vi "Execute.vi"(5 "SleepTerminalArray":refnum<vi>, 6 "ExeRef":refnum<vi>, 7 "ActiveTerminalArray":refnum<vi>, 8 "error in (no error)":errorcluster, 9 "Json_In":string, 10 "VariableRef":T2, 11 "Info":T1) -> (0 "Error Out":errorcluster, 1 "NumResultArray":dbl[](array[numeric]), 2 "StrResultArray":string[](array[string]), 3 "StrResult":string, 4 "NumResult":dbl)   [LabVIEW 2018, in "Number.lvlib"]
uses:
  Number.lvlib
  <userlib>/_OpenG.lib/dictionary/dictionary.llb/Dictionary Object RefNum__ogtk.ctl
  <userlib>/_OpenG.lib/dictionary/dictionary.llb/Dictionary Object RefNum - Enum__ogtk.ctl
  <vilib>/addons/_JKI.lib/Serialization/JSON/JKI JSON Serialization.lvlib
  <vilib>/gmath/NI_Gmath.lvlib
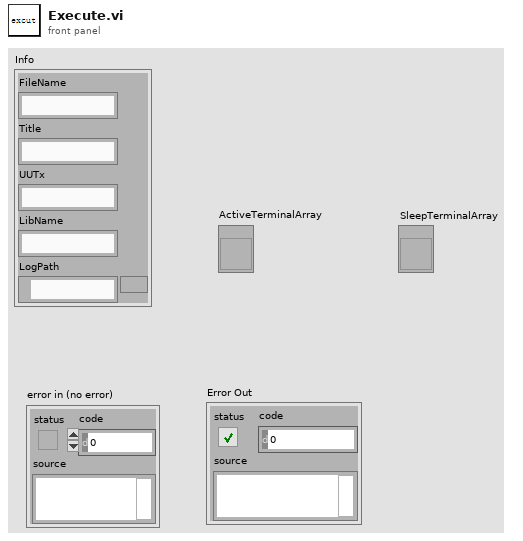
[diagram p1: front panel]
types:
  T1 = cluster{"FileName":string, "Title":string, "UUTx":string, "LibName":string, "LogPath":path}
  T2 = typedef "Dictionary Object RefNum__ogtk.ctl" = refnum<k1>
  T3 = cluster{"InitialNumber":cluster{"json":cluster{"Method":string, "InitialNum":dbl}}, "RandomNumber":cluster{"json":cluster{"Method":string, "Seed":dbl}}, "CalculateNumber":cluster{"json":cluster{"Method":string, "Type":string, "NumxVar":string, "NumyVar":string, "Formula":string}}, "CompareNumber":cluster{"json":cluster{"Method":string, "Type":string, "NumxVar":string, "NumyVar":string}}}
  T4 = cluster{"json":cluster{"Method":string, "InitialNum":dbl}}
  T5 = cluster{"json":cluster{"Method":string, "Seed":dbl}}
  T6 = cluster{"json":cluster{"Method":string, "Type":string, "NumxVar":string, "NumyVar":string, "Formula":string}}
  T7 = cluster{"json":cluster{"Method":string, "Type":string, "NumxVar":string, "NumyVar":string}}
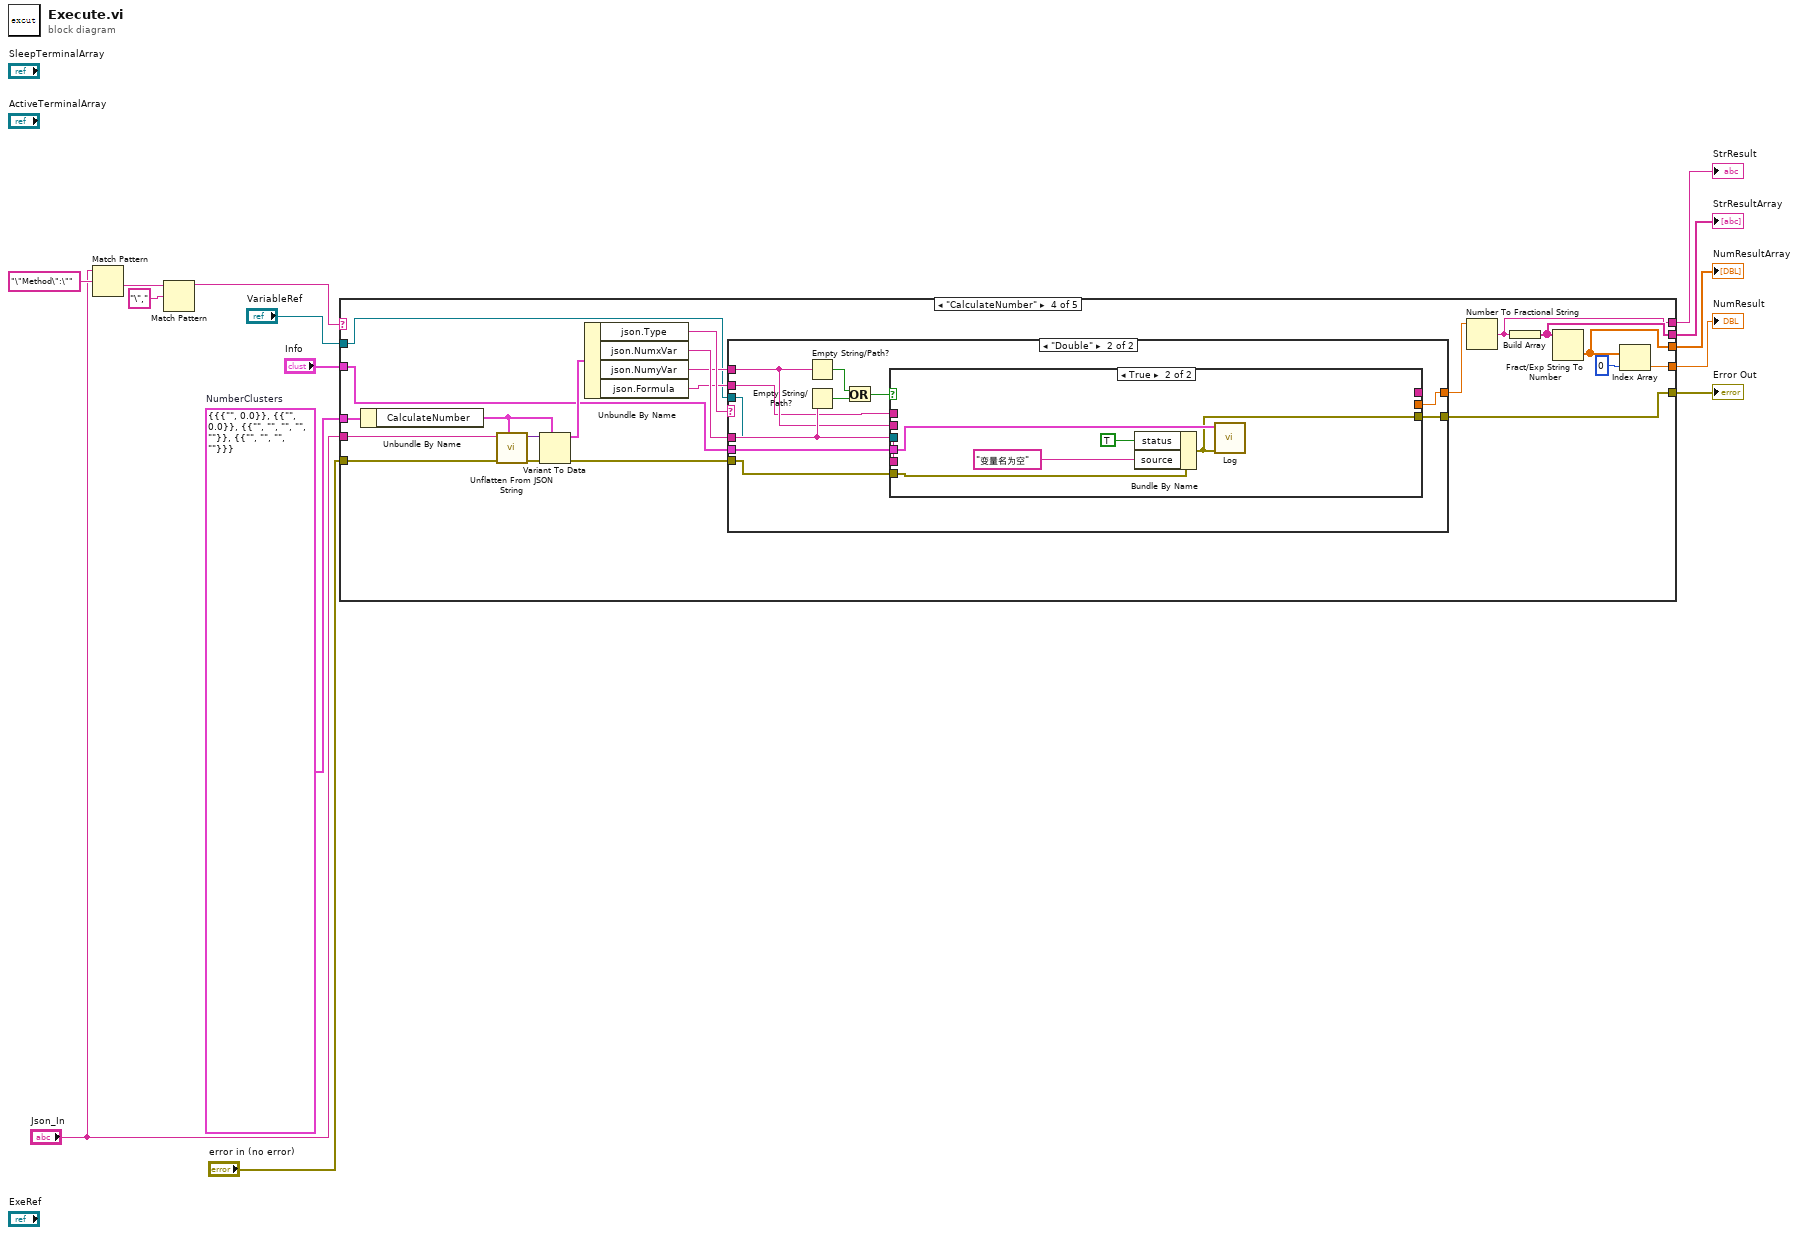
[diagram p0: block diagram]
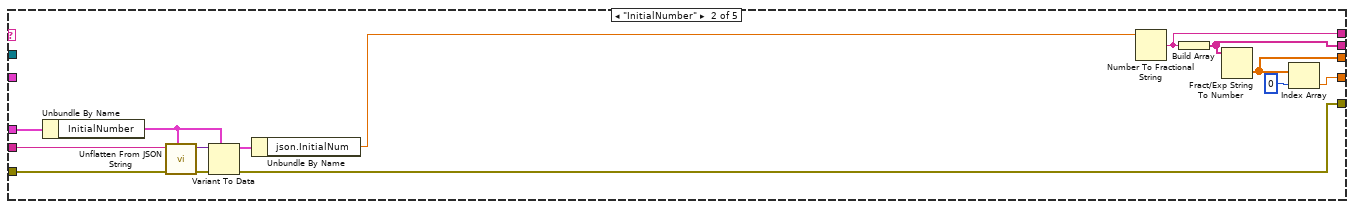
[diagram p3: hidden frame]
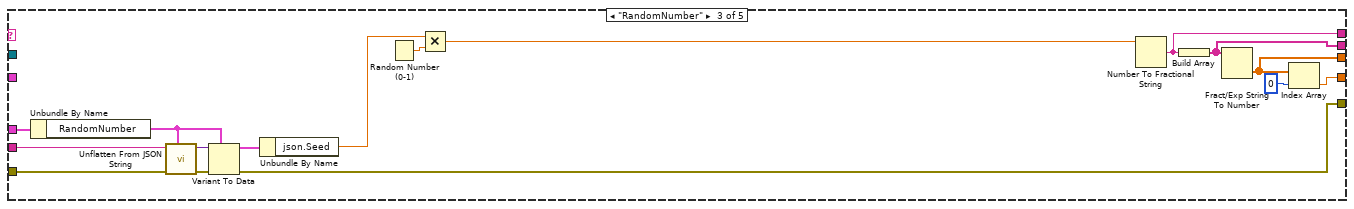
[diagram p4: hidden frame]
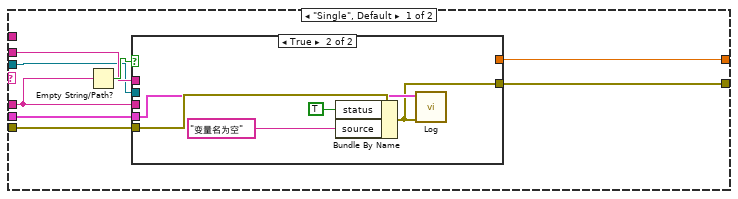
[diagram p5: hidden frame]
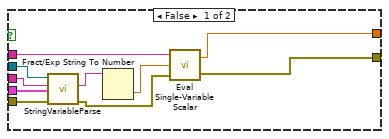
[diagram p6: hidden frame]
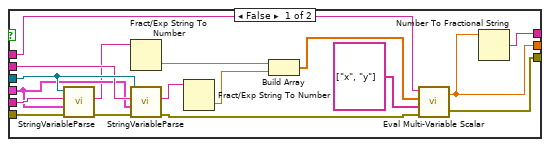
[diagram p7: hidden frame]
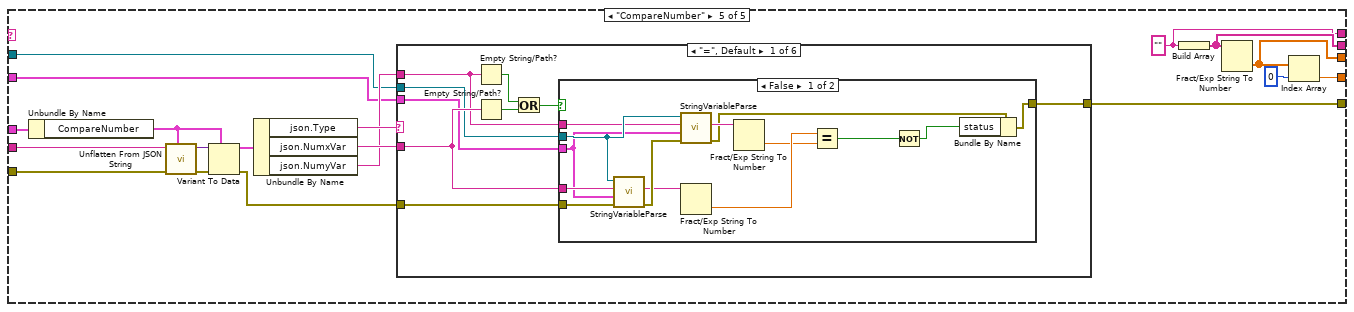
[diagram p8: hidden frame]
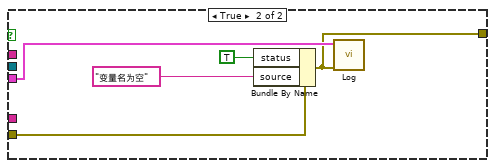
[diagram p9: hidden frame]
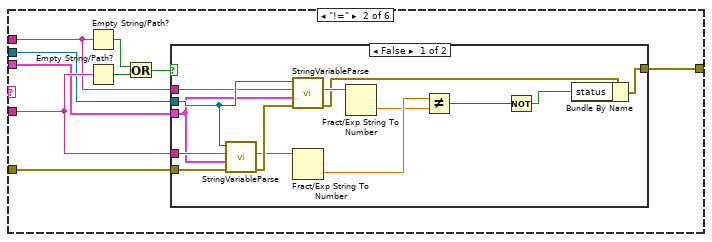
[diagram p10: hidden frame]
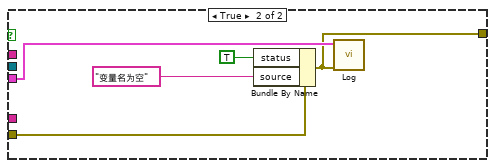
[diagram p11: hidden frame]
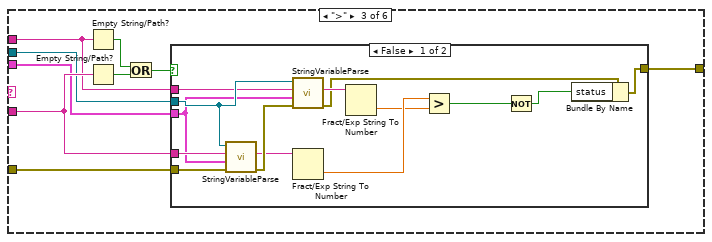
[diagram p12: hidden frame]
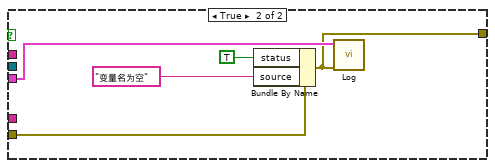
[diagram p13: hidden frame]
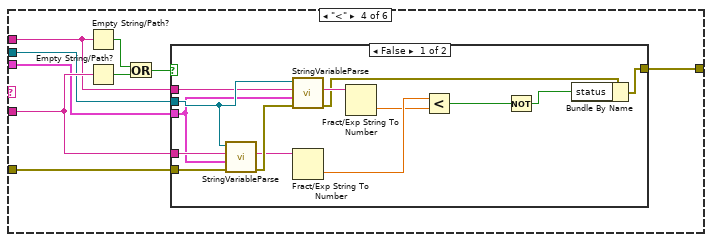
[diagram p14: hidden frame]
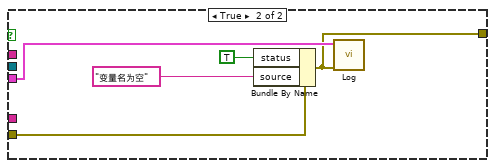
[diagram p15: hidden frame]
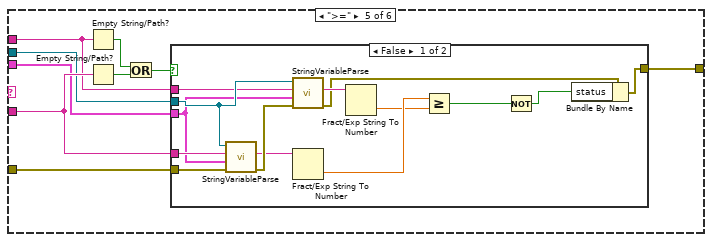
[diagram p16: hidden frame]
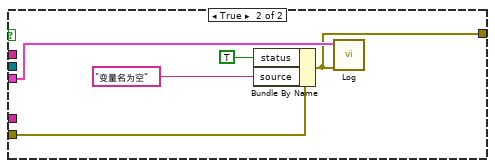
[diagram p17: hidden frame]
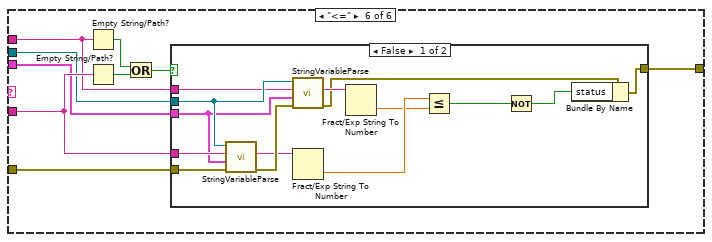
[diagram p18: hidden frame]
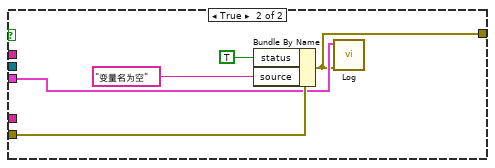
[diagram p19: hidden frame]
diagram:
  w1 = T3 {"InitialNumber"={"json"={"Method"="", "InitialNum"=0.0}}, "RandomNumber"={"json"={"Method"="", "Seed"=0.0}}, "CalculateNumber"={"json"={"Method"="", "Type"="", "NumxVar"="", "NumyVar"="", "Formula"=""}}, "CompareNumber"={"json"={"Method"="", "Type"="", "NumxVar"="", "NumyVar"=""}}}  # NumberClusters
  n1 = Match Pattern(string="Json_In", regular expression="\"Method\":\"") -> (after substring=w4:string)  [unwired: 1 in, 3 out]
  n2 = Match Pattern(string=w4, regular expression="\",") -> (before substring=w2:string)  [unwired: 1 in, 3 out]
  n3 = case shown="\"CalculateNumber\"" w2 {
    tunnel: "Json_In" -> [_ w26 w42 w63 w138]
    tunnel: [w15 w18 w34 w46 w124] -> w14
    tunnel: "error in (no error)" -> [w15 w25 w41 w62 w137]
    tunnel: [_ w17 w33 w47 w123] -> w12
    tunnel: "VariableRef" -> [_ _ _ w49 w125]
    tunnel: [_ w16 w32 w56 w131] -> w11
    tunnel: [_ w21 w37 w59 w134] -> w10
    tunnel: [_ w23 w39 w61 w136] -> w9
    tunnel: "Info" -> [_ _ _ w50 w126]
    tunnel: w1 -> [_ w20 w36 w58 w133]
    frame Default {
    }
    frame "InitialNumber" {
      n4 = Unbundle By Name(w20) -> ("InitialNumber"=w19:T4)
      n5 = call <vilib>:"Unflatten From JSON String.vi"("Type and Defaults"=w19, "error in (no error)"=w25, "JSON String"=w26) -> ("error out"=w28:errorcluster, "Variant"=w29:variant)  [unwired: 7 in]
      n6 = Variant To Data(error in=w28, type=w19, Variant=w29) -> (data=w27:T4, error out=w18:errorcluster)
      n7 = Unbundle By Name(w27) -> ("json.InitialNum"=w24:dbl)
      n8 = Number To Fractional String(number=w24) -> (F-format string=w17:string)  [unwired: 3 in]
      n9 = Build Array(w17) -> (w16:string[])
      n10 = Fract/Exp String To Number(string=w16) -> (number=w23:dbl[])  [unwired: 3 in, 1 out]
      n11 = Index Array(array=w23, index=0) -> (element=w21:dbl)
    }
    frame "RandomNumber" {
      n12 = Unbundle By Name(w36) -> ("RandomNumber"=w35:T5)
      n13 = call <vilib>:"Unflatten From JSON String.vi"("Type and Defaults"=w35, "error in (no error)"=w41, "JSON String"=w42) -> ("error out"=w44:errorcluster, "Variant"=w45:variant)  [unwired: 7 in]
      n14 = Variant To Data(error in=w44, type=w35, Variant=w45) -> (data=w43:T5, error out=w34:errorcluster)
      n15 = Unbundle By Name(w43) -> ("json.Seed"=w40:dbl)
      n16 = Random Number (0-1)() -> (number: 0 to 1=w30:dbl)
      n17 = Multiply(x=w40, y=w30) -> (x*y=w31:dbl)
      n18 = Number To Fractional String(number=w31) -> (F-format string=w33:string)  [unwired: 3 in]
      n19 = Build Array(w33) -> (w32:string[])
      n20 = Fract/Exp String To Number(string=w32) -> (number=w39:dbl[])  [unwired: 3 in, 1 out]
      n21 = Index Array(array=w39, index=0) -> (element=w37:dbl)
    }
    frame "CalculateNumber" {
      n22 = Unbundle By Name(w58) -> ("CalculateNumber"=w57:T6)
      n23 = call <vilib>:"Unflatten From JSON String.vi"("Type and Defaults"=w57, "error in (no error)"=w62, "JSON String"=w63) -> ("error out"=w65:errorcluster, "Variant"=w66:variant)  [unwired: 7 in]
      n24 = Variant To Data(error in=w65, type=w57, Variant=w66) -> (data=w64:T6, error out=w54:errorcluster)
      n25 = Unbundle By Name(w64) -> ("json.Type"=w55:string, "json.NumxVar"=w53:string, "json.NumyVar"=w52:string, "json.Formula"=w51:string)
      n26 = case shown="\"Double\"" w55 {
        tunnel: w54 -> [w74 w100]
        tunnel: [w73 w99] -> w46
        tunnel: w53 -> [w72 w98]
        tunnel: [w71 w97] -> w48
        tunnel: w52 -> [_ w93]
        tunnel: w51 -> [w69 w92]
        tunnel: w50 -> [w68 w91]
        tunnel: w49 -> [w67 w90]
        frame "Single", Default {
          n27 = Empty String/Path?(string/path=w72) -> (empty?=w70:bool)
          n28 = case shown="True" w70 {
            tunnel: w74 -> [w78 w89]
            tunnel: [w84 w85] -> w73
            tunnel: w72 -> [w79 _]
            tunnel: [w81 _] -> w71
            tunnel: w69 -> [w83 _]
            tunnel: w68 -> [w75 w87]
            tunnel: w67 -> [w80 _]
            frame False {
              n29 = call "StringVariableParse.vi"("error in"=w78, "Info"=w75, "in"=w79, "dictionary"=w80) -> ("error out"=w77:errorcluster, "out"=w76:string)  [unwired: 5 in, 1 out]
              n30 = Fract/Exp String To Number(string=w76) -> (number=w82:dbl)  [unwired: 3 in, 1 out]
              n31 = call <vilib>:"Eval Single-Variable Scalar.vi"("error in (no error)"=w77, "x value"=w82, "formula"=w83) -> ("error out"=w84:errorcluster, "y value"=w81:dbl)
            }
            frame True {
              n32 = Bundle By Name(cluster=w89, "status"=TRUE, "source"="变量名为空") -> (w85:errorcluster)
              n33 = call "Log.vi"("error in"=w85, "Info"=w87) -> ()  [unwired: 10 in]
            }
          }
        }
        frame "Double" {
          n34 = Empty String/Path?(string/path=w93) -> (empty?=w94:bool)
          n35 = Empty String/Path?(string/path=w98) -> (empty?=w96:bool)
          n36 = Or(x=w94, y=w96) -> (x .or. y?=w95:bool)
          n37 = case shown="True" w95 {
            tunnel: w100 -> [w105 w122]
            tunnel: [w112 w118] -> w99
            tunnel: w98 -> [w109 _]
            tunnel: [w110 _] -> _
            tunnel: [w111 _] -> w97
            tunnel: w93 -> [w107 _]
            tunnel: w92 -> [w117 _]
            tunnel: w91 -> [w106 w119]
            tunnel: w90 -> [w108 _]
            frame False {
              n38 = call "StringVariableParse.vi"("error in"=w105, "Info"=w106, "in"=w109, "dictionary"=w108) -> ("error out"=w104:errorcluster, "out"=w101:string)  [unwired: 5 in, 1 out]
              n39 = Fract/Exp String To Number(string=w101) -> (number=w115:dbl)  [unwired: 3 in, 1 out]
              n40 = call "StringVariableParse.vi"("error in"=w104, "Info"=w106, "in"=w107, "dictionary"=w108) -> ("error out"=w103:errorcluster, "out"=w102:string)  [unwired: 5 in, 1 out]
              n41 = Fract/Exp String To Number(string=w102) -> (number=w114:dbl)  [unwired: 3 in, 1 out]
              n42 = Build Array(w115, w114) -> (w113:dbl[])
              n43 = call <vilib>:"Eval Multi-Variable Scalar.vi"("error in (no error)"=w103, "Variables"=string[] ["x", "y"], "X Values"=w113, "formula"=w117) -> ("error out"=w112:errorcluster, "y value"=w111:dbl)
              n44 = Number To Fractional String(number=w111) -> (F-format string=w110:string)  [unwired: 3 in]
            }
            frame True {
              n45 = Bundle By Name(cluster=w122, "status"=TRUE, "source"="变量名为空") -> (w118:errorcluster)
              n46 = call "Log.vi"("error in"=w118, "Info"=w119) -> ()  [unwired: 10 in]
            }
          }
        }
      }
      n47 = Number To Fractional String(number=w48) -> (F-format string=w47:string)  [unwired: 3 in]
      n48 = Build Array(w47) -> (w56:string[])
      n49 = Fract/Exp String To Number(string=w56) -> (number=w61:dbl[])  [unwired: 3 in, 1 out]
      n50 = Index Array(array=w61, index=0) -> (element=w59:dbl)
    }
    frame "CompareNumber" {
      w123 = ""
      n51 = Unbundle By Name(w133) -> ("CompareNumber"=w132:T7)
      n52 = call <vilib>:"Unflatten From JSON String.vi"("Type and Defaults"=w132, "error in (no error)"=w137, "JSON String"=w138) -> ("error out"=w140:errorcluster, "Variant"=w141:variant)  [unwired: 7 in]
      n53 = Variant To Data(error in=w140, type=w132, Variant=w141) -> (data=w139:T7, error out=w129:errorcluster)
      n54 = Unbundle By Name(w139) -> ("json.Type"=w130:string, "json.NumxVar"=w128:string, "json.NumyVar"=w127:string)
      n55 = case shown="\"=\", Default" w130 {
        tunnel: w129 -> [w150 w178 w206 w234 w262 w290]
        tunnel: [w149 w177 w205 w233 w261 w289] -> w124
        tunnel: w128 -> [w148 w176 w204 w232 w260 w288]
        tunnel: w127 -> [w144 w172 w200 w228 w256 w284]
        tunnel: w126 -> [w143 w171 w199 w227 w255 w283]
        tunnel: w125 -> [w142 w170 w198 w226 w254 w282]
        frame "=", Default {
          n56 = Empty String/Path?(string/path=w144) -> (empty?=w145:bool)
          n57 = Empty String/Path?(string/path=w148) -> (empty?=w147:bool)
          n58 = Or(x=w145, y=w147) -> (x .or. y?=w146:bool)
          n59 = case shown="False" w146 {
            tunnel: w150 -> [w160 w169]
            tunnel: [w153 w165] -> w149
            tunnel: w148 -> [w164 _]
            tunnel: w144 -> [w162 _]
            tunnel: w143 -> [w161 w166]
            tunnel: w142 -> [w163 _]
            frame False {
              n60 = call "StringVariableParse.vi"("error in"=w160, "Info"=w161, "in"=w164, "dictionary"=w163) -> ("error out"=w159:errorcluster, "out"=w157:string)  [unwired: 5 in, 1 out]
              n61 = call "StringVariableParse.vi"("error in"=w159, "Info"=w161, "in"=w162, "dictionary"=w163) -> ("error out"=w152:errorcluster, "out"=w158:string)  [unwired: 5 in, 1 out]
              n62 = Fract/Exp String To Number(string=w157) -> (number=w156:dbl)  [unwired: 3 in, 1 out]
              n63 = Fract/Exp String To Number(string=w158) -> (number=w155:dbl)  [unwired: 3 in, 1 out]
              n64 = Equal?(x=w156, y=w155) -> (x = y?=w151:bool)
              n65 = Not(x=w151) -> (.not. x?=w154:bool)
              n66 = Bundle By Name(cluster=w152, "status"=w154) -> (w153:errorcluster)
            }
            frame True {
              n67 = Bundle By Name(cluster=w169, "status"=TRUE, "source"="变量名为空") -> (w165:errorcluster)
              n68 = call "Log.vi"("error in"=w165, "Info"=w166) -> ()  [unwired: 10 in]
            }
          }
        }
        frame "!=" {
          n69 = Empty String/Path?(string/path=w172) -> (empty?=w173:bool)
          n70 = Empty String/Path?(string/path=w176) -> (empty?=w175:bool)
          n71 = Or(x=w173, y=w175) -> (x .or. y?=w174:bool)
          n72 = case shown="False" w174 {
            tunnel: w178 -> [w188 w197]
            tunnel: [w181 w193] -> w177
            tunnel: w176 -> [w192 _]
            tunnel: w172 -> [w190 _]
            tunnel: w171 -> [w189 w194]
            tunnel: w170 -> [w191 _]
            frame False {
              n73 = call "StringVariableParse.vi"("error in"=w188, "Info"=w189, "in"=w192, "dictionary"=w191) -> ("error out"=w187:errorcluster, "out"=w185:string)  [unwired: 5 in, 1 out]
              n74 = call "StringVariableParse.vi"("error in"=w187, "Info"=w189, "in"=w190, "dictionary"=w191) -> ("error out"=w180:errorcluster, "out"=w186:string)  [unwired: 5 in, 1 out]
              n75 = Fract/Exp String To Number(string=w185) -> (number=w184:dbl)  [unwired: 3 in, 1 out]
              n76 = Fract/Exp String To Number(string=w186) -> (number=w183:dbl)  [unwired: 3 in, 1 out]
              n77 = Not Equal?(x=w184, y=w183) -> (x != y?=w179:bool)
              n78 = Not(x=w179) -> (.not. x?=w182:bool)
              n79 = Bundle By Name(cluster=w180, "status"=w182) -> (w181:errorcluster)
            }
            frame True {
              n80 = Bundle By Name(cluster=w197, "status"=TRUE, "source"="变量名为空") -> (w193:errorcluster)
              n81 = call "Log.vi"("error in"=w193, "Info"=w194) -> ()  [unwired: 10 in]
            }
          }
        }
        frame ">" {
          n82 = Empty String/Path?(string/path=w200) -> (empty?=w201:bool)
          n83 = Empty String/Path?(string/path=w204) -> (empty?=w203:bool)
          n84 = Or(x=w201, y=w203) -> (x .or. y?=w202:bool)
          n85 = case shown="False" w202 {
            tunnel: w206 -> [w216 w225]
            tunnel: [w209 w221] -> w205
            tunnel: w204 -> [w220 _]
            tunnel: w200 -> [w218 _]
            tunnel: w199 -> [w217 w222]
            tunnel: w198 -> [w219 _]
            frame False {
              n86 = call "StringVariableParse.vi"("error in"=w216, "Info"=w217, "in"=w220, "dictionary"=w219) -> ("error out"=w215:errorcluster, "out"=w213:string)  [unwired: 5 in, 1 out]
              n87 = call "StringVariableParse.vi"("error in"=w215, "Info"=w217, "in"=w218, "dictionary"=w219) -> ("error out"=w208:errorcluster, "out"=w214:string)  [unwired: 5 in, 1 out]
              n88 = Fract/Exp String To Number(string=w213) -> (number=w212:dbl)  [unwired: 3 in, 1 out]
              n89 = Fract/Exp String To Number(string=w214) -> (number=w211:dbl)  [unwired: 3 in, 1 out]
              n90 = Greater?(x=w212, y=w211) -> (0:w207:bool)
              n91 = Not(x=w207) -> (.not. x?=w210:bool)
              n92 = Bundle By Name(cluster=w208, "status"=w210) -> (w209:errorcluster)
            }
            frame True {
              n93 = Bundle By Name(cluster=w225, "status"=TRUE, "source"="变量名为空") -> (w221:errorcluster)
              n94 = call "Log.vi"("error in"=w221, "Info"=w222) -> ()  [unwired: 10 in]
            }
          }
        }
        frame "<" {
          n95 = Empty String/Path?(string/path=w228) -> (empty?=w229:bool)
          n96 = Empty String/Path?(string/path=w232) -> (empty?=w231:bool)
          n97 = Or(x=w229, y=w231) -> (x .or. y?=w230:bool)
          n98 = case shown="False" w230 {
            tunnel: w234 -> [w244 w253]
            tunnel: [w237 w249] -> w233
            tunnel: w232 -> [w248 _]
            tunnel: w228 -> [w246 _]
            tunnel: w227 -> [w245 w250]
            tunnel: w226 -> [w247 _]
            frame False {
              n99 = call "StringVariableParse.vi"("error in"=w244, "Info"=w245, "in"=w248, "dictionary"=w247) -> ("error out"=w243:errorcluster, "out"=w241:string)  [unwired: 5 in, 1 out]
              n100 = call "StringVariableParse.vi"("error in"=w243, "Info"=w245, "in"=w246, "dictionary"=w247) -> ("error out"=w236:errorcluster, "out"=w242:string)  [unwired: 5 in, 1 out]
              n101 = Fract/Exp String To Number(string=w241) -> (number=w240:dbl)  [unwired: 3 in, 1 out]
              n102 = Fract/Exp String To Number(string=w242) -> (number=w239:dbl)  [unwired: 3 in, 1 out]
              n103 = Less?(x=w240, y=w239) -> (x < y?=w235:bool)
              n104 = Not(x=w235) -> (.not. x?=w238:bool)
              n105 = Bundle By Name(cluster=w236, "status"=w238) -> (w237:errorcluster)
            }
            frame True {
              n106 = Bundle By Name(cluster=w253, "status"=TRUE, "source"="变量名为空") -> (w249:errorcluster)
              n107 = call "Log.vi"("error in"=w249, "Info"=w250) -> ()  [unwired: 10 in]
            }
          }
        }
        frame ">=" {
          n108 = Empty String/Path?(string/path=w256) -> (empty?=w257:bool)
          n109 = Empty String/Path?(string/path=w260) -> (empty?=w259:bool)
          n110 = Or(x=w257, y=w259) -> (x .or. y?=w258:bool)
          n111 = case shown="False" w258 {
            tunnel: w262 -> [w272 w281]
            tunnel: [w265 w277] -> w261
            tunnel: w260 -> [w276 _]
            tunnel: w256 -> [w274 _]
            tunnel: w255 -> [w273 w278]
            tunnel: w254 -> [w275 _]
            frame False {
              n112 = call "StringVariableParse.vi"("error in"=w272, "Info"=w273, "in"=w276, "dictionary"=w275) -> ("error out"=w271:errorcluster, "out"=w269:string)  [unwired: 5 in, 1 out]
              n113 = call "StringVariableParse.vi"("error in"=w271, "Info"=w273, "in"=w274, "dictionary"=w275) -> ("error out"=w264:errorcluster, "out"=w270:string)  [unwired: 5 in, 1 out]
              n114 = Fract/Exp String To Number(string=w269) -> (number=w268:dbl)  [unwired: 3 in, 1 out]
              n115 = Fract/Exp String To Number(string=w270) -> (number=w267:dbl)  [unwired: 3 in, 1 out]
              n116 = Greater Or Equal?(x=w268, y=w267) -> (x >= y?=w263:bool)
              n117 = Not(x=w263) -> (.not. x?=w266:bool)
              n118 = Bundle By Name(cluster=w264, "status"=w266) -> (w265:errorcluster)
            }
            frame True {
              n119 = Bundle By Name(cluster=w281, "status"=TRUE, "source"="变量名为空") -> (w277:errorcluster)
              n120 = call "Log.vi"("error in"=w277, "Info"=w278) -> ()  [unwired: 10 in]
            }
          }
        }
        frame "<=" {
          n121 = Empty String/Path?(string/path=w284) -> (empty?=w285:bool)
          n122 = Empty String/Path?(string/path=w288) -> (empty?=w287:bool)
          n123 = Or(x=w285, y=w287) -> (x .or. y?=w286:bool)
          n124 = case shown="False" w286 {
            tunnel: w290 -> [w300 w309]
            tunnel: [w293 w305] -> w289
            tunnel: w288 -> [w304 _]
            tunnel: w284 -> [w302 _]
            tunnel: w283 -> [w301 w306]
            tunnel: w282 -> [w303 _]
            frame False {
              n125 = call "StringVariableParse.vi"("error in"=w300, "Info"=w301, "in"=w304, "dictionary"=w303) -> ("error out"=w299:errorcluster, "out"=w297:string)  [unwired: 5 in, 1 out]
              n126 = call "StringVariableParse.vi"("error in"=w299, "Info"=w301, "in"=w302, "dictionary"=w303) -> ("error out"=w292:errorcluster, "out"=w298:string)  [unwired: 5 in, 1 out]
              n127 = Fract/Exp String To Number(string=w297) -> (number=w296:dbl)  [unwired: 3 in, 1 out]
              n128 = Fract/Exp String To Number(string=w298) -> (number=w295:dbl)  [unwired: 3 in, 1 out]
              n129 = Less Or Equal?(x=w296, y=w295) -> (x <= y?=w291:bool)
              n130 = Not(x=w291) -> (.not. x?=w294:bool)
              n131 = Bundle By Name(cluster=w292, "status"=w294) -> (w293:errorcluster)
            }
            frame True {
              n132 = Bundle By Name(cluster=w309, "status"=TRUE, "source"="变量名为空") -> (w305:errorcluster)
              n133 = call "Log.vi"("error in"=w305, "Info"=w306) -> ()  [unwired: 10 in]
            }
          }
        }
      }
      n134 = Build Array(w123) -> (w131:string[])
      n135 = Fract/Exp String To Number(string=w131) -> (number=w136:dbl[])  [unwired: 3 in, 1 out]
      n136 = Index Array(array=w136, index=0) -> (element=w134:dbl)
    }
  }
  "StrResult" <- w12
  "Error Out" <- w14
  "StrResultArray" <- w11
  "NumResult" <- w10
  "NumResultArray" <- w9
